vi "SubVI_Gain_Conversion.vi"(11 "Amp commands":u8[][](array[numeric])) -> (3 "Gain Weights":i32[](array[numeric]))   [LabVIEW 2020]
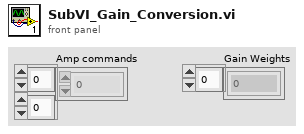
[diagram p1: front panel]
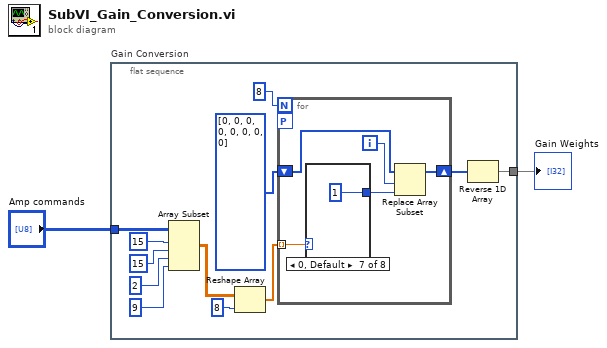
[diagram p0: block diagram]
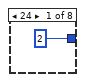
[diagram p2: hidden frame]
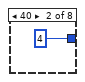
[diagram p3: hidden frame]
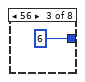
[diagram p4: hidden frame]
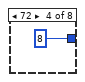
[diagram p5: hidden frame]
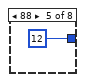
[diagram p6: hidden frame]
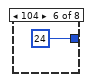
[diagram p7: hidden frame]
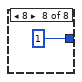
[diagram p8: hidden frame]
diagram:
  n1 = flat-sequence "Gain Conversion" {
    tunnel: "Amp commands" -> [w5]
    tunnel: [w3] -> w1
    frame #0 {
      n2 = Array Subset(array=w5, index (row)=15 ("row 1"), length (row)=15 ("row N"), index (col)=2 ("column 1"), length (col)=9 ("column N")) -> (w10:dbl[][])
      n3 = Reshape Array(w10, 8 ("dimension size")) -> (w13:dbl[])
      n4 = for {
        N: 8 -> [_]
        tunnel: w13 -> [w15] mode=indexing
        shift-right: [w17] -> w14
        shift-left: i32[] [0, 0, 0, 0, 0, 0, 0, 0] -> [w19]
        workers-P: _ -> [_]
        i -> [w18]
        n5 = case shown="0, Default" w15 {
          tunnel: [2 4 6 8 12 24 1 1] -> w16
          frame 24 {
          }
          frame 40 {
          }
          frame 56 {
          }
          frame 72 {
          }
          frame 88 {
          }
          frame 104 {
          }
          frame 0, Default {
          }
          frame 8 {
          }
        }
        n6 = Replace Array Subset(array=w19, new element=w16, index=w18) -> (w17:i32[])
      }
      n7 = Reverse 1D Array(array=w14) -> (reversed array=w3:i32[])
    }
  }
  "Gain Weights" <- w1
